vi "TurnOff.vi"(8 "error in (no error)":errorcluster, 11 "OutDoorLight in":refnum<class "OutDoorLight.lvclass">) -> (0 "error out":errorcluster, 3 "OutDoorLight out":refnum<class "OutDoorLight.lvclass">)   [LabVIEW 2013, in "OutDoorLight.lvclass"]
uses:
  OutDoorLight.lvclass
  OutDoorLight.lvclass/OutDoorLight.ctl
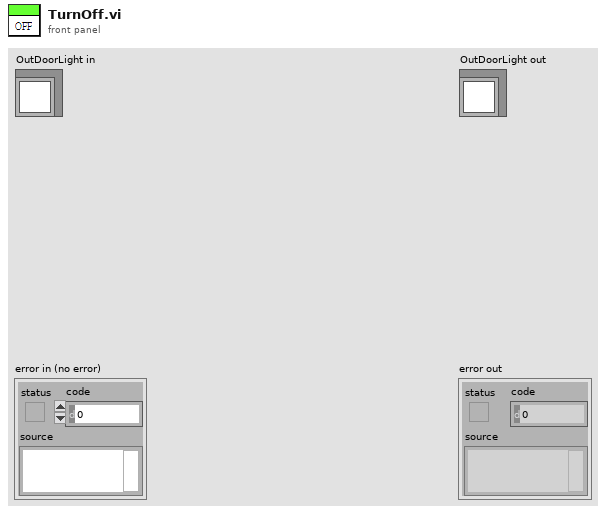
[diagram p1: front panel]
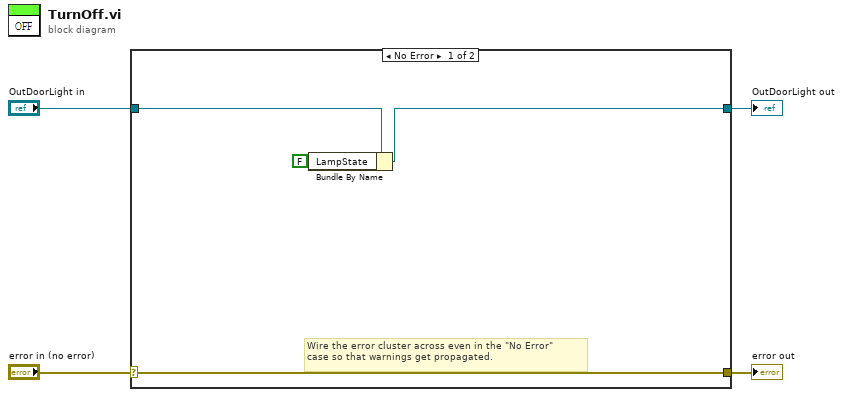
[diagram p0: block diagram]
diagram:
  n1 = case shown="No Error" "error in (no error)" {
    selector: "error in (no error)" -> [w8 w10]
    tunnel: [w8 w10] -> w3
    tunnel: [w6 w9] -> w1
    tunnel: "OutDoorLight in" -> [w7 w9]
    frame No Error {
      # "Wire the error cluster across even in the \"No Error\"\ncase so that warnings get propagated."
      n2 = Bundle By Name(cluster=w7, "LampState"=FALSE ("TurnON")) -> (w6:refnum<class "OutDoorLight.lvclass">)
    }
    frame Error {
    }
  }
  "error out" <- w3
  "OutDoorLight out" <- w1
